vi "Initialize SCARA Serial Arm.vi"(8 "error in (no error)":errorcluster, 10 "offsets":dbl[](array[numeric])=[0.0, 0.0, 0.0, 0.0], 11 "lengths":dbl[](array[numeric])) -> (0 "error out":errorcluster, 3 "SCARA serial arm out":refnum<class "NI_Robotics_SCARA Serial Arm Class.lvclass">)   [LabVIEW 2017, in "NI_Robotics_SCARA Serial Arm Class.lvclass"]
doc: "Sets the properties of a serial robot arm and generates a representation of the arm. If you have access to a 6R, 5R, or SCARA arm, generate that type of arm. If you do not have access to an arm of those types, generate a generic arm. You must manually select the polymorphic instance to use."
uses:
  <vilib>/robotics/Kinematics/Analytical/SCARA/NI_Robotics_SCARA Serial Arm Class.lvclass
  c:/Program Files (x86)/National Instruments/LabVIEW 2017/vi.lib/robotics/Kinematics/Robot/NI_Robotics_Serial Robot Arm.lvclass
  <vilib>/robotics/Kinematics/Analytical/SCARA/NI_Robotics_SCARA Serial Arm Class.lvclass/NI_Robotics_SCARA Serial Arm Class.ctl
  <vilib>/robotics/Kinematics/DH Kinematic Parameters.ctl
  <vilib>/robotics/Kinematics/Link/Joint Type.ctl
  <vilib>/robotics/Kinematics/Link/NI_Robotics_Link.lvclass
  <vilib>/robotics/Kinematics/Robot/NI_Robotics_Serial Robot Arm.lvclass
  <vilib>/robotics/Utilities/NI_Robotics Utilities.lvlib
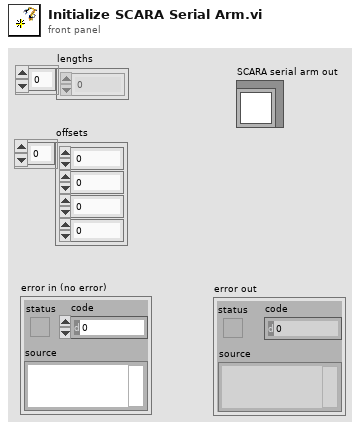
[diagram p1: front panel]
types:
  T1 = typedef "NI_Robotics_Link.lvclass/Joint Type.ctl" = enum16{"Revolute", "Prismatic"}
  T2 = typedef "DH Kinematic Parameters.ctl" = cluster{"twist angle":dbl, "length":dbl, "rotation angle":dbl, "offset distance":dbl, "joint type":T1, "joint coordinate offset":dbl}
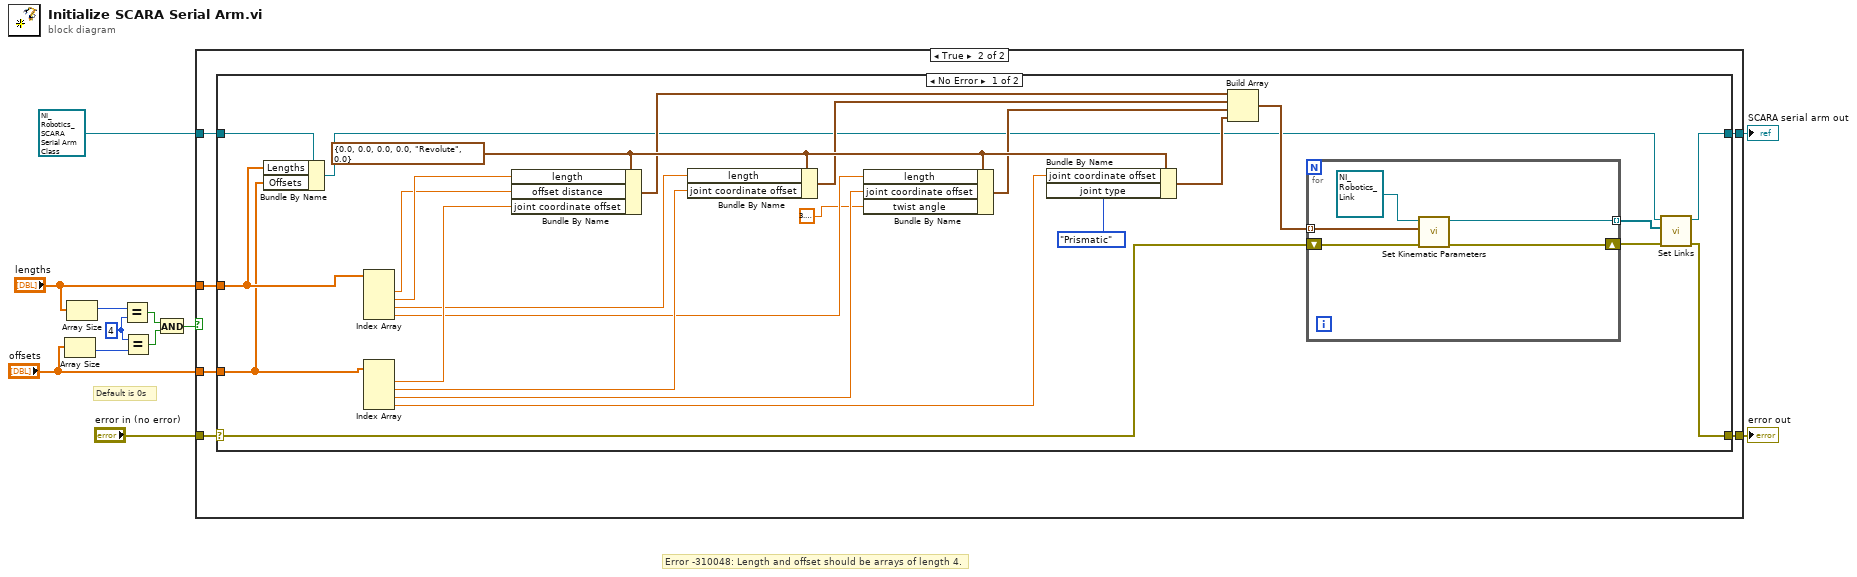
[diagram p0: block diagram]
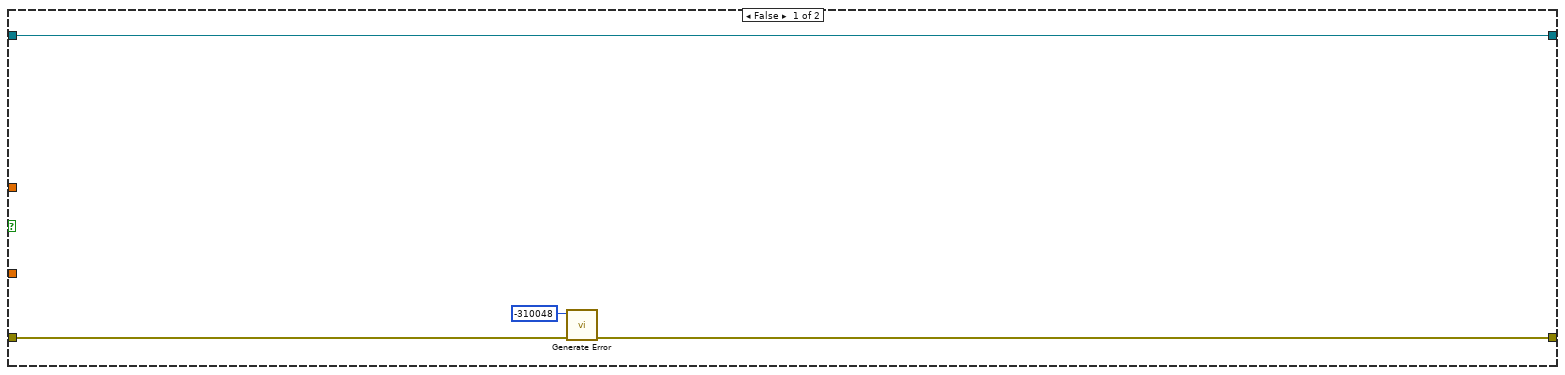
[diagram p2: hidden frame]
diagram:
  w4 = 4 ("y")
  # "Error -310048: Length and offset should be arrays of length 4."
  # "Default is 0s"
  n1 = Array Size(array="offsets") -> (size(s)=w5:i32)
  n2 = Array Size(array="lengths") -> (size(s)=w6:i32)
  n3 = Equal?(x=w6, y=w4) -> (x = y?=w3:bool)
  n4 = Equal?(x=w4, y=w5) -> (x = y?=w2:bool)
  n5 = And(x=w3, y=w2) -> (x .and. y?=w1:bool)
  n6 = case shown="True" w1 {
    tunnel: "error in (no error)" -> [w15 w22]
    tunnel: [w14 w21] -> w11
    tunnel: [w16 w20] -> w10
    tunnel: refnum<class "NI_Robotics_SCARA Serial Arm Class.lvclass"> refnum ("SCARA Serial Arm Class in") -> [w16 w19]
    tunnel: "lengths" -> [_ w18]
    tunnel: "offsets" -> [_ w17]
    frame False {
      n7 = call <vilib>:"Generate Error.vi"("error in (no error)"=w15, "code"=-310048) -> ("error out"=w14:errorcluster)  [unwired: 9 in]
    }
    frame True {
      n8 = case shown="No Error" w22 {
        selector: w22 -> [w23 w54]
        tunnel: [w24 w54] -> w21
        tunnel: [w27 w53] -> w20
        tunnel: w19 -> [w32 w53]
        tunnel: w18 -> [w31 _]
        tunnel: w17 -> [w30 _]
        frame No Error {
          w47 = T2 {"twist angle"=0.0, "length"=0.0, "rotation angle"=0.0, "offset distance"=0.0, "joint type"=enum."Revolute", "joint coordinate offset"=0.0} ("Link Parameters")
          n9 = Bundle By Name(cluster=w32, "Lengths"=w31, "Offsets"=w30) -> (w28:refnum<class "NI_Robotics_SCARA Serial Arm Class.lvclass">)
          n10 = Index Array(array=w31) -> (element #1=w41:dbl, element #2=w42:dbl, element #3=w39:dbl, element #4=w37:dbl)  [unwired: 4 in]
          n11 = Index Array(array=w30) -> (element #1=w40:dbl, element #2=w38:dbl, element #3=w36:dbl, element #4=w33:dbl)  [unwired: 4 in]
          n12 = Bundle By Name(cluster=w47, "length"=w42, "offset distance"=w41, "joint coordinate offset"=w40) -> (w43:T2)
          n13 = Bundle By Name(cluster=w47, "length"=w39, "joint coordinate offset"=w38) -> (w44:T2)
          n14 = Bundle By Name(cluster=w47, "length"=w37, "joint coordinate offset"=w36, "twist angle"=3.141592653589793) -> (w45:T2)
          n15 = Bundle By Name(cluster=w47, "joint coordinate offset"=w33, "joint type"=Joint_Type."Prismatic" ("Joint Type")) -> (w46:T2)
          n16 = Build Array(w43, w44, w45, w46) -> (w29:T2[])
          n17 = for {
            tunnel: w29 -> [w51] mode=indexing
            tunnel: [w49] -> w26 mode=indexing
            shift-right: [w48] -> w25
            shift-left: w23 -> [w50]
            n18 = call <vilib>:"Set Kinematic Parameters.vi"("error in (no error)"=w50, "kinematic parameters"=w51, "link in"=refnum<class "NI_Robotics_Link.lvclass"> refnum ("Link")) -> ("error out"=w48:errorcluster, "link out"=w49:refnum<class "NI_Robotics_Link.lvclass">)  [unwired: 7 in]
          }
          n19 = call <vilib>:"Set Links.vi"("error in (no error)"=w25, "links"=w26, "serial arm in"=w28) -> ("error out"=w24:errorcluster, "serial arm out"=w27:refnum<class "NI_Robotics_SCARA Serial Arm Class.lvclass">)  [unwired: 7 out]
        }
        frame Error {
        }
      }
    }
  }
  "error out" <- w11
  "SCARA serial arm out" <- w10
